vi "PH_PP_CurrentMeas.constructor.vi"(0 "name":string, 2 "data in":string, 5 "error in(no error)":errorcluster) -> (14 "i ref out":refnum<vi>, 16 "data out":string, 19 "error out":errorcluster)   [LabVIEW 2014, in "PH_PP_CurrentMeas.lvlib"]
doc: "This class is forseen to get and indicate the data of the current measurement of the pulsed power at PHELIX. For this purpose it acts on instances of PPMA_DAQClient.\n\nThis class is part of the PHELIX user layer.\n\nauthor: Stefan Götte, GSI\n\nLicense Agreement for this software:\n\nCopyright (C)\nGesellschaft für Schwerionenforschung, GSI\nPlanckstr. 1\n64291 Darmstadt\nGermany\n\nContact: D.Beck@gsi.de \n\nThis program is free software; you can redistribute it and/or modify it under the terms of the \nGNU General Public License as published by the Free Software Foundation; either version 2 of \nthe license, or (at your option) any later version.\n\nThis program is distributed in the hope that it will be useful, but WITHOUT ANY WARRANTY; \nwithout even the implied warranty of MERCHANTABILITY or FITNESS FOR A PARTICULAR PURPOSE. See the GNU General License for more details (http://www.gnu.org).\n\nGesellschaft für Schwerionenforschung, GSI\nPlanckstr. 1, 64291 Darmstadt, Germany\nFor all questions and ideas contact: M.Richter@gsi.de, H.Brand@gsi.de or D.Beck@gsi.de.\nLast update: 16-JUN-2004"
uses:
  PH_PP_CurrentMeas.lvlib
  PH_Basics/PH_PSDBWriter/PH_PSDBWriter.lvlib
  CS_Core/CSObj/CSObj.lvlib
  PH_Basics/PH_Class/PH_Class.lvlib
  PH_Basics/PH_StatusHandler/PH_StatusHandler.lvlib
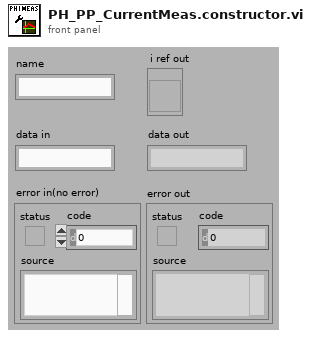
[diagram p1: front panel]
types:
  T1 = enum16{"SetAttribute", "GetAttribute", "CreateAttribute", "DestroyAttribute", "DestroyAllAtributes"}
  T2 = typedef "PH_PP_CurrentMeas.lvlib/PH_PP_CurrentMeas.i attribute.ctl" = cluster{"Status":cluster{"GUI Ref Hardware Feedback":refnum<vi>, "Tab Control":refnum<vi>}, "PU 1":cluster{"Instance":string, "Status":T3, "Ref Status ":refnum<vi>, "Data":waveform(dbl)[], "Ref Data":refnum<vi>}, "PU 2":cluster{"Instance":string, "Status":T3, "Ref Status ":refnum<vi>, "Data":waveform(dbl)[], "Ref Data":refnum<vi>}, "PU 3":cluster{"Instance":string, "Status":T3, "Ref Status ":refnum<vi>, "Data":waveform(dbl)[], "Ref Data":refnum<vi>}, "PU 4":cluster{"Instance":string, "Status":T3, "Ref Status ":refnum<vi>, "Data":waveform(dbl)[], "Ref Data":refnum<vi>}, "PU 5":cluster{"Instance":string, "Status":T3, "Ref Status ":refnum<vi>, "Data":waveform(dbl)[], "Ref Data":refnum<vi>}, "FR":cluster{"Instance":string, "Status":T3, "Ref Status ":refnum<vi>, "Data":waveform(dbl)[], "Ref Data":refnum<vi>}, "PA - 19mm 1":cluster{"Instance":string, "Status":T3, "Ref Status ":refnum<vi>}, "PA - 19mm 2":cluster{"Instance":string, "Status":T3, "Ref Status ":refnum<vi>, "no link":bool}, "PA - 45mm":cluster{"Instance":string, "Status":T3, "Ref Status ":refnum<vi>, "no link":bool}, "PA Data":cluster{"Data":waveform(dbl)[], "Ref":refnum<vi>}, "Sequencer":cluster{"Instance":string, "SM State Ref":refnum<vi>}, "Tasks":cluster{"Port":u16, "connection ID":refnum<k5>, "Status":T3, "Ref":refnum<vi>, "Ref Bar":refnum<vi>, "Feedback":cluster{"Received Data Sets":T4[], "Driver Error":errorcluster, "Connection not established":bool, "Error unpacking the data":bool, "No Task defined":bool, "Not triggered yet":bool}, "Data":waveform(dbl)[], "Ref Teststart Task":refnum<vi>}[], "in use":cluster{"MA DP":bool, "FR and PA":bool}, "DAQ Server":string}
  T3 = typedef "PH_StatusHandler.lvlib/PH_StatusHandler.Status.ctl" = i16
  T4 = typedef "PH_PP_CurrentMeas.lvlib/PH_PP_CurrentMeas.CommandCluster.ctl" = cluster{"Command":string, "Data":string, "error out":errorcluster}
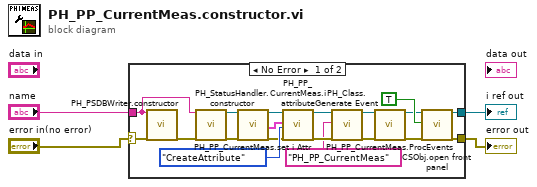
[diagram p0: block diagram]
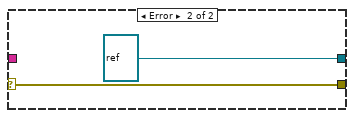
[diagram p2: hidden frame]
diagram:
  n1 = case shown="No Error" "error in(no error)" {
    selector: "error in(no error)" -> [w8 w25]
    tunnel: [w23 w25] -> w4
    tunnel: [w22 refnum<vi> refnum ("i ref out")] -> w3
    tunnel: "name" -> [w5 _]
    frame No Error {
      n2 = call "PH_PSDBWriter.constructor.vi"("name"=w5, "error in"=w8) -> ("error out"=w18:errorcluster)  [unwired: 15 in, 2 out]
      n3 = call "PH_StatusHandler.constructor.vi"("name"=w5, "error in(no error)"=w18) -> ("i ref out"=w6:refnum<vi>, "error out"=w7:errorcluster)  [unwired: 15 in, 1 out]
      n4 = call "PH_PP_CurrentMeas.set i Attr.vi"("i ref in"=w6, "error in (no error)"=w7) -> ("i ref out"=w17:refnum<vi>, "i Attributes"=w20:T2, "error out"=w16:errorcluster)  [unwired: 15 in]
      n5 = call "PH_PP_CurrentMeas.i attribute.vi"("VI Refnum"=w17, "CLASS.i attribute"=w20, "Action"=T1."CreateAttribute", "error in (no error)"=w16) -> ("VI Refnum out"=w15:refnum<vi>, "error out"=w14:errorcluster)  [unwired: 13 in, 1 out]
      n6 = call "PH_Class.Generate Event.vi"("i ref in"=w15, "Class"="PH_PP_CurrentMeas", "error in (no error)"=w14) -> ("i ref out"=w13:refnum<vi>, "error out"=w12:errorcluster)  [unwired: 15 in]
      n7 = call "PH_PP_CurrentMeas.ProcEvents.vi"("i ref in"=w13, "error in"=w12) -> ("i ref out"=w10:refnum<vi>, "error out"=w9:errorcluster)  [unwired: 16 in]
      n8 = call "CSObj.open front panel.vi"("i ref in"=w10, "frontPanelOpen"=TRUE, "error in (no error)"=w9) -> ("i ref out"=w22:refnum<vi>, "error out"=w23:errorcluster)  [unwired: 15 in]
    }
    frame Error {
    }
  }
  "i ref out" <- w3
  "error out" <- w4
